vi "XSFP_18BackTo17.vi"(10 "Version-State Cluster In":T1, 11 "XRef":refnum<vi>) -> (0 "Custom Label":string, 1 "Custom Warning To Issue":string, 2 "Version-State Cluster Out":T1, 3 "Action":T2)   [LabVIEW 2020]
uses:
  <vilib>/XSFPSupport/SFPChangeStateAction.ctl
  <vilib>/XNodeSupport/XNodeVersion.ctl
  <vilib>/XNodeSupport/XNodeUShort.ctl
  <vilib>/XSFPSupport/NI_XSFPSupport.lvlib
  <vilib>/XNodeSupport/NI_XNodeSupport.lvlib
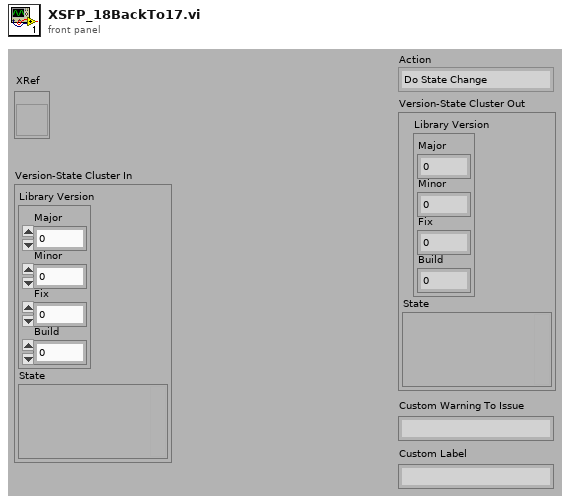
[diagram p1: front panel]
types:
  T1 = cluster{"Library Version":cluster{"Major":u16, "Minor":u16, "Fix":u16, "Build":u16}, "State":variant}
  T2 = typedef "NI_XSFPSupport.lvlib/SFPChangeStateAction.ctl" = enum32{"Do State Change", "Replace With Label", "Fail SFP"}
  T3 = typedef "NI_XNodeSupport.lvlib/XNodeVersion.ctl" = cluster{"Major":T4, "Minor":T4, "Fix":T4, "Build":T4}
  T4 = typedef "NI_XNodeSupport.lvlib/XNodeUShort.ctl" = u16
  T5 = cluster{"Major":u16, "Minor":u16, "Fix":u16, "Build":u16}
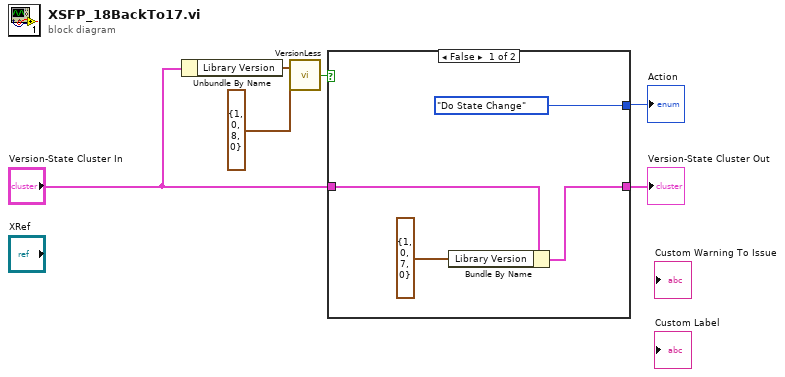
[diagram p0: block diagram]
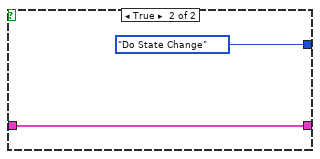
[diagram p2: hidden frame]
diagram:
  n1 = Unbundle By Name("Version-State Cluster In") -> ("Library Version"=w1:T5)
  n2 = call <vilib>:"VersionLess.vi"("y"=T3 {"Major"=1, "Minor"=0, "Fix"=8, "Build"=0}, "x"=w1) -> ("x < y?"=w6:bool)
  n3 = case shown="False" w6 {
    tunnel: [SFPChangeStateAction."Do State Change" ("Action") SFPChangeStateAction."Do State Change" ("Action")] -> w5
    tunnel: [w10 w11] -> w4
    tunnel: "Version-State Cluster In" -> [w8 w11]
    frame False {
      n4 = Bundle By Name(cluster=w8, "Library Version"=T3 {"Major"=1, "Minor"=0, "Fix"=7, "Build"=0} ("y")) -> (w10:T1)
    }
    frame True {
    }
  }
  "Action" <- w5
  "Version-State Cluster Out" <- w4
